vi "NI_FPGA_PPG.add service.vi"(0 "i ref in":refnum<vi>, 3 "ms timeout (10000)":i32=10000, 5 "error in (no error)":errorcluster) -> (14 "i ref out":refnum<vi>, 17 "timed out":bool, 19 "error out":errorcluster)   [LabVIEW 2014, in "NI_FPGA_PPG.lvlib"]
doc: "Creates 2 DIM services.\n\nLicense Agreement for this software:\n\nCopyright (C) 2009\nFalk Ziegler\nInstitut für Physik\nErnst-Moritz-Arndt Universität\nFelix-Hausdorff-Str. 6\n17487 Greifswald\n\nContact: Falk Ziegler, ziegler@physik.uni-greifswald.de\n\nThis program is free software: you can redistribute it and/or modify it under the terms of the GNU General Public License as published by the Free Software Foundation, either version 3 of the License, or (at your option) any later version.\n\nThis program is distributed in the hope that it will be useful, but WITHOUT ANY WARRANTY; without even the implied warranty of MERCHANTABILITY or FITNESS FOR A PARTICULAR PURPOSE. See the GNU General Public License for more details.\n\nYou should have received a copy of the GNU General Public License along with this program. If not, see <http://www.gnu.org/licenses/>.\n\nFor all questions and ideas contact: ziegler@physik.uni-greifswald.de or d.beck@gsi.de\nLast update: 01-Sep-2009"
uses:
  NI_FPGA_PPG.lvlib
  CSCore/CSSystem/CSSystemLib/CSSystemLib.lvlib
  CSlibraries-extern/DimLVEvent/LVDimInterface/LVDimInterface.lvlib
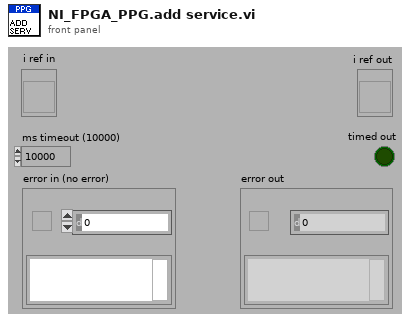
[diagram p1: front panel]
types:
  T1 = typedef "NI_FPGA_PPG.lvlib/NI_FPGA_PPG.i attribute.ctl" = cluster{"dim_service_id":cluster{"dim_actual_device_status":i32, "dim_event_data":i32, "dim_cmd_data":i32, "dim_cmd_data _description":i32, "dim_channel_description":i32}, "VISA":refnum<visa-resource-name>, "actual_device_status":i32, "event_data_id":i32, "pdc_enabled":bool, "pdc_timestamp":u32, "cmd_data_string":string, "cmd_data_size":i32, "cmd_data_description_string":string, "cmd_data_description_size":i32, "channel_description_string":string, "channel_description_size":i32}
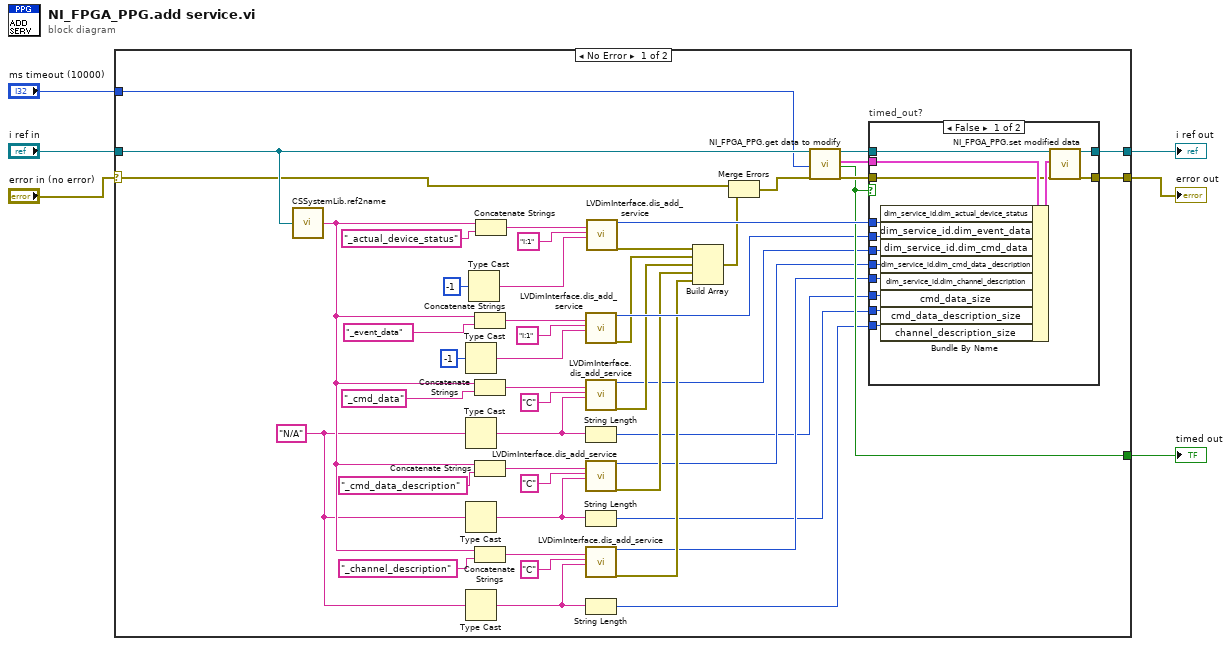
[diagram p0: block diagram]
diagram:
  n1 = case shown="No Error" "error in (no error)" {
    selector: "error in (no error)" -> [w35 w71]
    tunnel: "i ref in" -> [w49 w72]
    tunnel: [w46 w72] -> w4
    tunnel: [w47 w71] -> w3
    tunnel: "ms timeout (10000)" -> [w42 _]
    tunnel: [w41 _] -> w1
    frame No Error {
      w10 = "N/A" ("substring (\"\")")
      n2 = call "CSSystemLib.ref2name.vi"("obj refnum"=w49) -> ("name"=w23:string)
      n3 = Type Cast(x=-1) -> (*(type *) &x=w36:string)  [unwired: 1 in]
      n4 = Type Cast(x=w10) -> (*(type *) &x=w13:string)  [unwired: 1 in]
      n5 = Type Cast(x=w10) -> (*(type *) &x=w12:string)  [unwired: 1 in]
      n6 = Type Cast(x=w10) -> (*(type *) &x=w11:string)  [unwired: 1 in]
      n7 = Type Cast(x=-1) -> (*(type *) &x=w54:string)  [unwired: 1 in]
      n8 = Concatenate Strings(w23, "_event_data" ("string")) -> (w38:string)
      n9 = Concatenate Strings(w23, "_cmd_data" ("string")) -> (w31:string)
      n10 = Concatenate Strings(w23, "_cmd_data_description" ("string")) -> (w28:string)
      n11 = Concatenate Strings(w23, "_channel_description" ("string")) -> (w25:string)
      n12 = Concatenate Strings(w23, "_actual_device_status" ("string")) -> (w52:string)
      n13 = call "LVDimInterface.dis_add_service.vi"("serviceName"=w38, "typeDescriptor"="I:1", "data"=w36) -> ("my_serviceID"=w33:i32, "error out"=w21:errorcluster)  [unwired: 15 in]
      n14 = call "LVDimInterface.dis_add_service.vi"("serviceName"=w31, "typeDescriptor"="C", "data"=w13) -> ("my_serviceID"=w16:i32, "error out"=w20:errorcluster)  [unwired: 15 in]
      n15 = String Length(string=w13) -> (length=w9:i32)
      n16 = call "LVDimInterface.dis_add_service.vi"("serviceName"=w28, "typeDescriptor"="C", "data"=w12) -> ("my_serviceID"=w15:i32, "error out"=w19:errorcluster)  [unwired: 15 in]
      n17 = String Length(string=w12) -> (length=w8:i32)
      n18 = call "LVDimInterface.dis_add_service.vi"("serviceName"=w25, "typeDescriptor"="C", "data"=w11) -> ("my_serviceID"=w14:i32, "error out"=w18:errorcluster)  [unwired: 15 in]
      n19 = String Length(string=w11) -> (length=w7:i32)
      n20 = call "LVDimInterface.dis_add_service.vi"("serviceName"=w52, "typeDescriptor"="I:1", "data"=w54) -> ("my_serviceID"=w44:i32, "error out"=w22:errorcluster)  [unwired: 15 in]
      n21 = Build Array(w22, w21, w20, w19, w18) -> (w17:errorcluster[])
      n22 = Merge Errors(w35, w17) -> (w34:errorcluster)
      n23 = call "NI_FPGA_PPG.get data to modify.vi"("i ref in"=w49, "ms timeout (10000)"=w42, "error in (no error)"=w34) -> ("i ref out"=w48:refnum<vi>, "i attribute"=w45:T1, "timed out"=w41:bool, "error out"=w43:errorcluster)  [unwired: 13 in]
      n24 = case "timed_out?" shown="False" w41 {
        tunnel: w48 -> [w68 w70]
        tunnel: [w67 w69] -> w47
        tunnel: [w66 w70] -> w46
        tunnel: w45 -> [w65 _]
        tunnel: w44 -> [w64 _]
        tunnel: w43 -> [w62 w69]
        tunnel: w33 -> [w61 _]
        tunnel: w16 -> [w60 _]
        tunnel: w15 -> [w59 _]
        tunnel: w14 -> [w58 _]
        tunnel: w9 -> [w57 _]
        tunnel: w8 -> [w56 _]
        tunnel: w7 -> [w55 _]
        frame False {
          n25 = Bundle By Name(cluster=w65, "dim_service_id.dim_actual_device_status"=w64, "dim_service_id.dim_event_data"=w61, "dim_service_id.dim_cmd_data"=w60, "dim_service_id.dim_cmd_data _description"=w59, "dim_service_id.dim_channel_description"=w58, "cmd_data_size"=w57, "cmd_data_description_size"=w56, "channel_description_size"=w55) -> (w63:T1)
          n26 = call "NI_FPGA_PPG.set modified data.vi"("i ref in"=w68, "i attribute"=w63, "error in (no error)"=w62) -> ("i ref out"=w66:refnum<vi>, "error out"=w67:errorcluster)  [unwired: 15 in]
        }
        frame True {
        }
      }
    }
    frame Error {
    }
  }
  "error out" <- w3
  "i ref out" <- w4
  "timed out" <- w1
